vi "ProcessCommand.vi"(5 "Ctl Refnum":refnum<vi>, 7 "Command":variant, 8 "error in (no error)":errorcluster, 9 "Data":T2=variant(string "Default"), 10 "Queue with Cluster Reference":T1, 11 "UserMenu Command in":refnum<class "UserMenu Command.lvclass">) -> (0 "error out":errorcluster, 2 "Queue (dup)":T1, 3 "UserMenu Command out":refnum<class "UserMenu Command.lvclass">)   [LabVIEW 2010, in "UserMenu Command.lvclass"]
uses:
  UserMenu Command.lvclass
  <userlib>/Common/Queue with Cluster/TYP_Queue with Cluster Reference.ctl
  Controls/TYP_VariantDefault.ctl
  UserMenu Command.lvclass/UserMenu Command.ctl
  <userlib>/Common/Queue with Cluster/Enqueue - ClusterBoth.vi
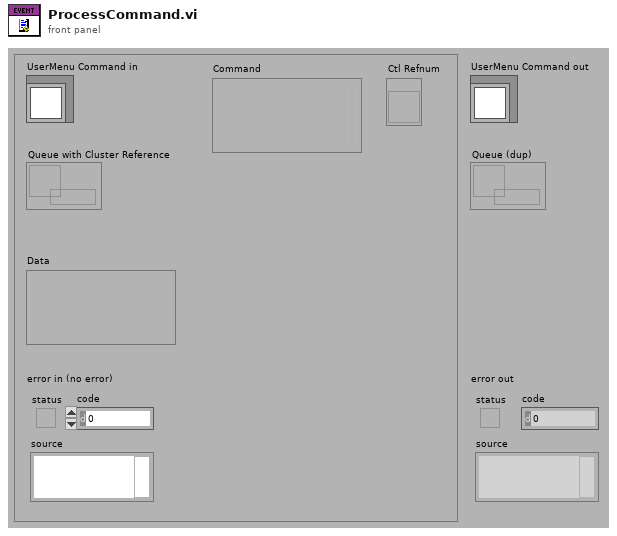
[diagram p1: front panel]
types:
  T1 = typedef "TYP_Queue with Cluster Reference.ctl" = refnum<queue>
  T2 = typedef "TYP_VariantDefault.ctl" = variant
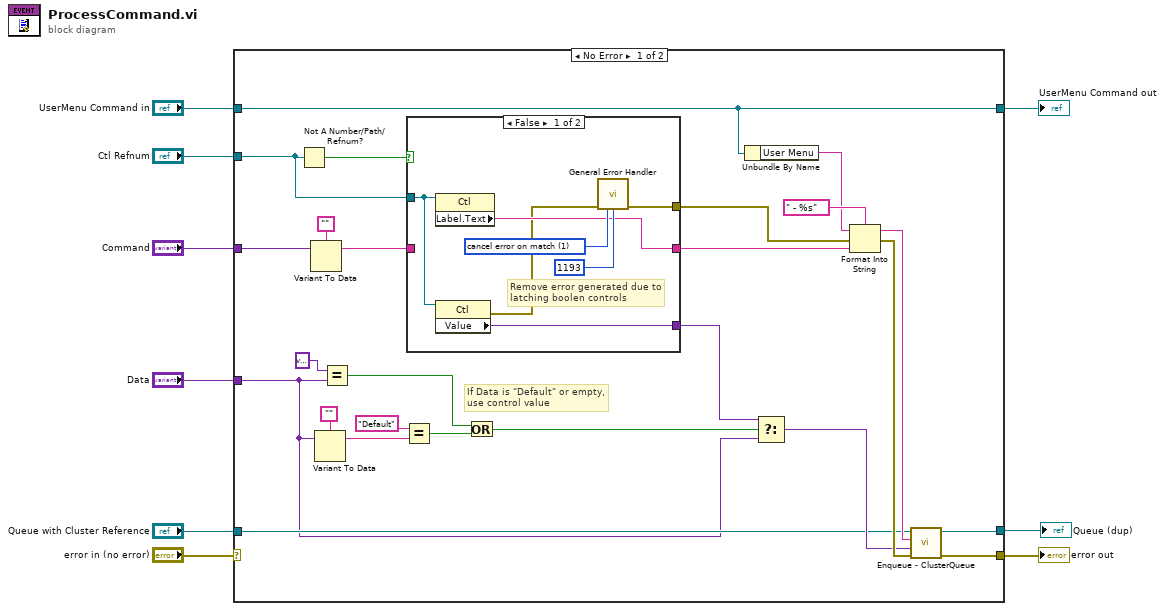
[diagram p0: block diagram]
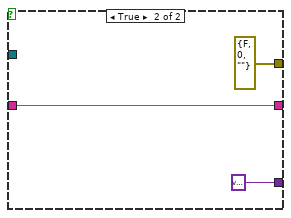
[diagram p2: hidden frame]
diagram:
  n1 = case shown="No Error" "error in (no error)" {
    selector: "error in (no error)" -> [_ w47]
    tunnel: [w16 w47] -> w8
    tunnel: [w14 w46] -> w6
    tunnel: "UserMenu Command in" -> [w14 w46]
    tunnel: "Queue with Cluster Reference" -> [w13 w45]
    tunnel: [w15 w45] -> w4
    tunnel: "Ctl Refnum" -> [w12 _]
    tunnel: "Data" -> [w11 _]
    tunnel: "Command" -> [w10 _]
    frame No Error {
      # "If Data is \"Default\" or empty,\nuse control value"
      n2 = Not A Number/Path/Refnum?(number/path/refnum=w12) -> (NaN/Path/Refnum?=w34:bool)
      n3 = Variant To Data(Variant=w10, type="") -> (data=w18:string)  [unwired: 1 in, 1 out]
      n4 = Variant To Data(Variant=w11, type="") -> (data=w25:string)  [unwired: 1 in, 1 out]
      n5 = Equal?(x=variant ("Value"), y=w11) -> (x = y?=w30:bool)
      n6 = Equal?(x="Default", y=w25) -> (x = y?=w31:bool)
      n7 = case shown="False" w34 {
        tunnel: w18 -> [_ w44]
        tunnel: [w37 w44] -> w21
        tunnel: [w40 variant ("Value")] -> w28
        tunnel: w12 -> [w36 _]
        tunnel: [w38 errorcluster {"status"=FALSE, "code"=0, "source"=""} ("error out")] -> w33
        frame False {
          w41 = 1 items=["no exception", "cancel error on match", "set error on match"] ("[exception action] (none:0)")
          # "Remove error generated due to\nlatching boolen controls"
          n8 = property class="Ctl"(reference=w36) -> ("Label.Text"=w37:string)  [unwired: 1 in, 2 out]
          n9 = property class="Ctl"(reference=w36) -> (error out=w35:errorcluster, "Value"=w40:variant)  [unwired: 1 in, 1 out]
          n10 = call <vilib>:"General Error Handler.vi"("error in (no error)"=w35, "[exception action] (none:0)"=w41, "[exception code]"=1193) -> ("error out"=w38:errorcluster)  [unwired: 8 in, 4 out]
        }
        frame True {
        }
      }
      n11 = Or(x=w30, y=w31) -> (x .or. y?=w32:bool)
      n12 = Unbundle By Name(w14) -> ("User Menu"=w19:string)
      n13 = Select(t=w28, s=w32, f=w11) -> (s? t:f=w24:T2)
      n14 = Format Into String(format string=" - %s", initial string=w19, error in=w33, w21) -> (resulting string=w22:string, error out=w27:errorcluster)
      n15 = call-poly <userlib>:"Enqueue - ClusterQueue.vi"("error in (no error)"=w27, "Data"=w24, "Command"=w22, "Queue with Cluster Reference"=w13) -> ("error out"=w16:errorcluster, "Queue Out (dup)"=w15:T1)  [unwired: 6 in]
    }
    frame Error {
    }
  }
  "error out" <- w8
  "UserMenu Command out" <- w6
  "Queue (dup)" <- w4
